vi "add-href.vi"(7 "State machine":T1=enum."add-icon-image-only", 10 "relative path":path) -> (2 "state":T2)   [LabVIEW 2014]
uses:
  controls/state program.ctl
  controls/state-machine.ctl
panel:
  in  "dummy":T2
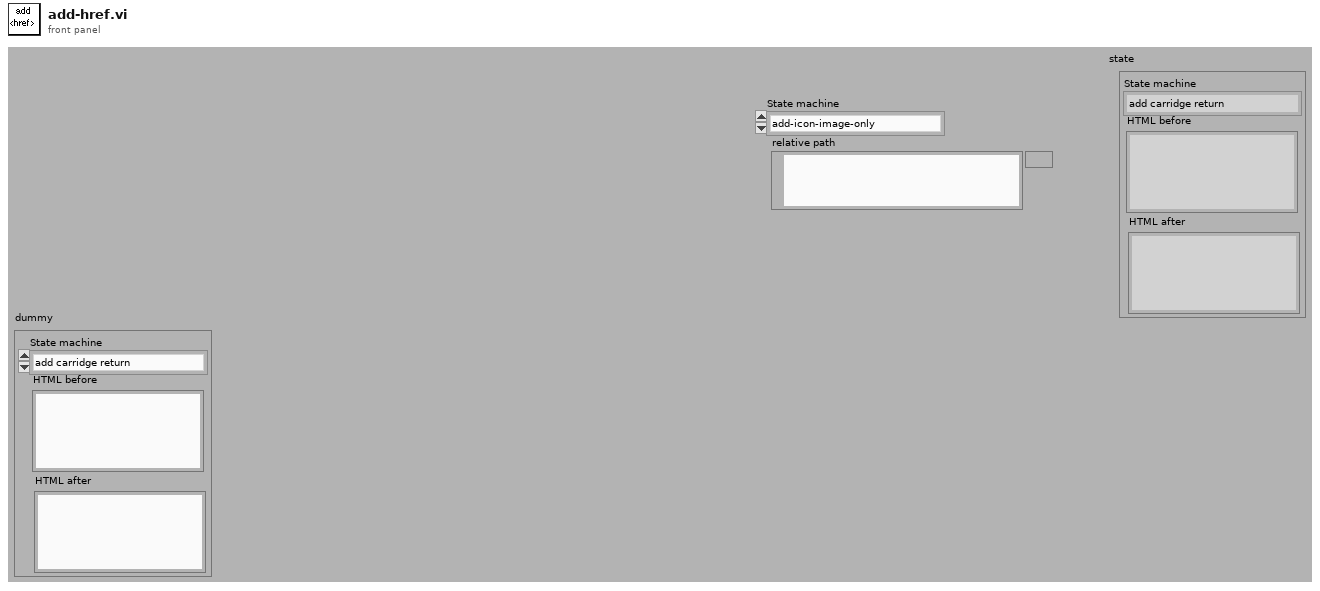
[diagram p1: front panel]
types:
  T1 = typedef "state-machine.ctl" = enum16{"add carridge return", "init", "Read-inputs", "edit generated file", "end", "Add front panel", "Add Block Diagram", "Add VI icon", "Add VI description", "Add VI hiearchy", "Add list of sub vis", "add custom html", "open report in browser", "Save report to file", "dispose report", "Add header text", "Create style .css", "add-red-box-header", "Delete Temp Files", "Remove-path-element", "add-revision-history", "add-icon-image-only"}
  T2 = typedef "state program.ctl" = cluster{"State machine":T1, "HTML before":string, "HTML after":string}
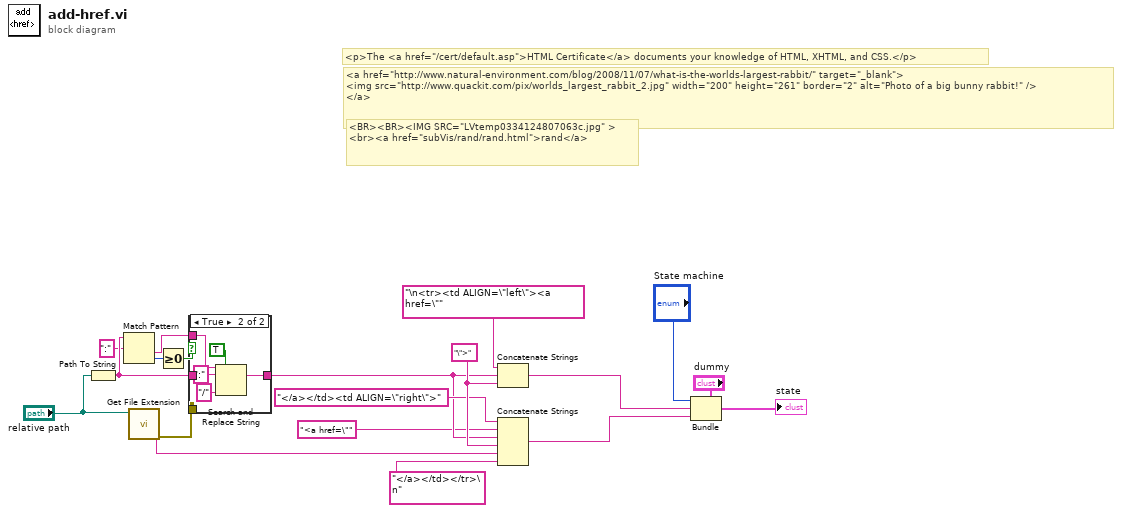
[diagram p0: block diagram]
diagram:
  w14 = "\">" ("string")
  # "<BR><BR><IMG SRC=\"LVtemp0334124807063c.jpg\" >\n<br><a href=\"subVis/rand/rand.html\">rand</a>"
  # "<a href=\"http://www.natural-environment.com/blog/2008/11/07/what-is-the-worlds-largest-rabbit/\" target=\"_blank\">\n<img src=\"http://www.quackit.com/pix/worlds_largest_rabbit_2.jpg\" width=\"200\" height=\"261\" border=\"2\" alt=\"Photo of a big bunny rabbit!\" />\n</a>"
  # "<p>The <a href=\"/cert/default.asp\">HTML Certificate</a> documents your knowledge of HTML, XHTML, and CSS.</p>"
  n1 = Path To String(path="relative path") -> (string=w10:string)
  n2 = Match Pattern(string=w10, regular expression=":") -> (after substring=w9:string, offset past match=w7:i32)  [unwired: 3 out]
  n3 = call <vilib>:"Get File Extension.vi"("file"="relative path") -> ("error out"=w2:errorcluster, "filename without extension"=w4:string)  [unwired: 1 in, 8 out]
  n4 = Greater Or Equal To 0?(x=w7) -> (x >= 0?=w8:bool)
  n5 = case shown="True" w8 {
    tunnel: [w20 w25] -> w3
    tunnel: w9 -> [_ w24]
    tunnel: w10 -> [w20 _]
    tunnel: w2 -> [_ _]
    frame False {
    }
    frame True {
      n6 = Search and Replace String(replace all?=TRUE ("replace all? (F)"), input string=w24, search string=":", replace string="/" ("replace string (\"\")")) -> (result string=w25:string)  [unwired: 1 in, 6 out]
    }
  }
  n7 = Concatenate Strings("\n<tr><td ALIGN=\"left\"><a href=\"", w3, w14) -> (w12:string)
  n8 = Concatenate Strings("</a></td><td ALIGN=\"right\">", "<a href=\"", w3, w14, w4, "</a></td></tr>\n") -> (w16:string)
  n9 = Bundle(cluster="dummy", "State machine"="State machine", "HTML before"=w12, "HTML after"=w16) -> (→"state":T2)
